vi "Example HistogramTrending.vi"() -> ()   [LabVIEW 2014]
uses:
  TrendingWithHistogramm.xctl
  <vilib>/ptbypt/NI_PtbyPt.lvlib
panel:
  out "TrendingWithHistogramm":dbl(xcontrol)
  in  "stop":bool
  in  "Mean":dbl
  in  "standard deviation":dbl=1.0 format="%0.2f"
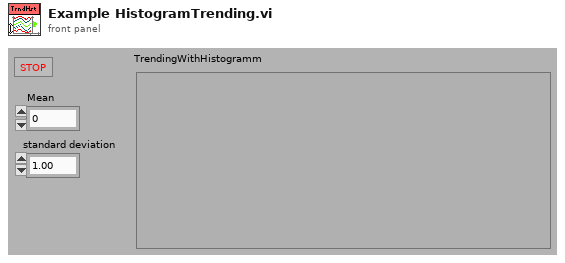
[diagram p1: front panel]
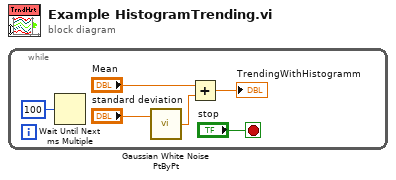
[diagram p0: block diagram]
diagram:
  n1 = while {
    stop <- "stop" stop-if-true
    n2 = Wait Until Next ms Multiple(millisecond multiple=u32 100) -> ()  [unwired: 1 out]
    n3 = call <vilib>:"Gaussian White Noise PtByPt.vi"("standard deviation"="standard deviation") -> ("Gaussian white noise"=w6:dbl)  [unwired: 2 in]
    n4 = Add(x="Mean", y=w6) -> (x+y=→"TrendingWithHistogramm":dbl)
  }
